vi "PV Software IGN State.vi"(11 "HEX Data (U8)":u8 format="%x") -> (3 "IGN State":string)   [LabVIEW 2023]
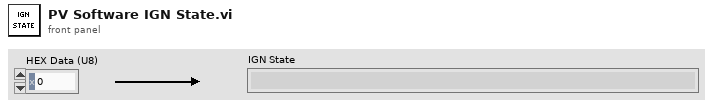
[diagram p1: front panel]
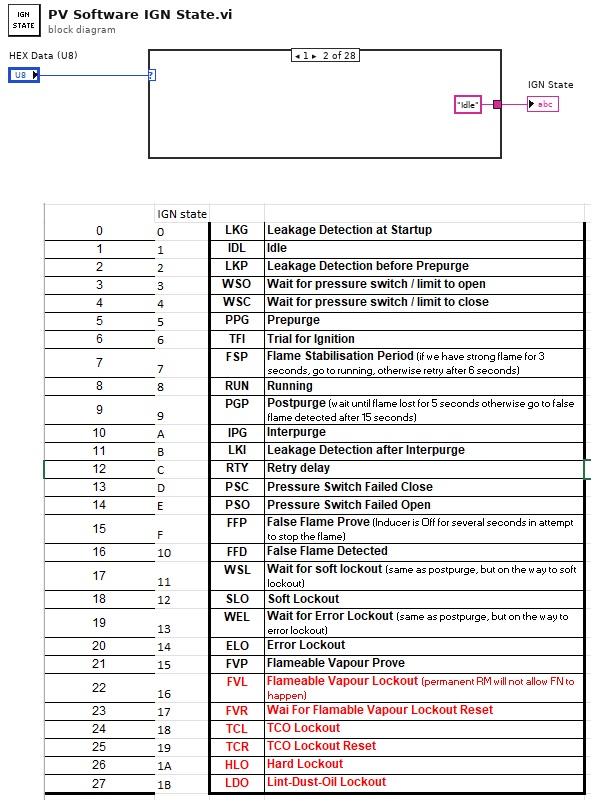
[diagram p0: block diagram]
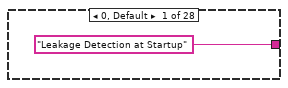
[diagram p2: hidden frame]
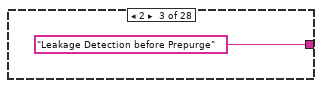
[diagram p3: hidden frame]
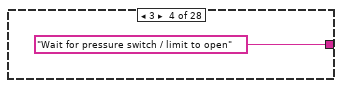
[diagram p4: hidden frame]
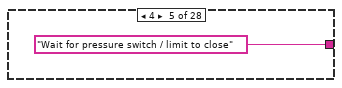
[diagram p5: hidden frame]
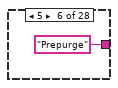
[diagram p6: hidden frame]
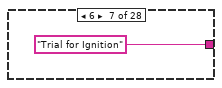
[diagram p7: hidden frame]
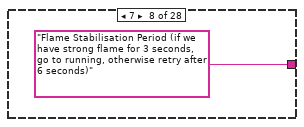
[diagram p8: hidden frame]
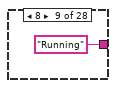
[diagram p9: hidden frame]
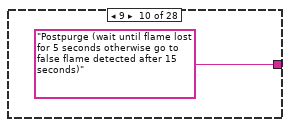
[diagram p10: hidden frame]
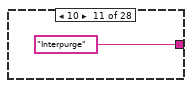
[diagram p11: hidden frame]
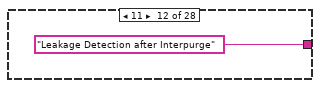
[diagram p12: hidden frame]
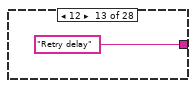
[diagram p13: hidden frame]
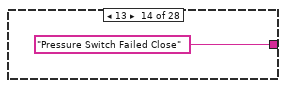
[diagram p14: hidden frame]
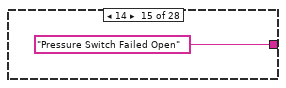
[diagram p15: hidden frame]
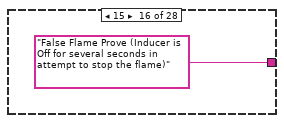
[diagram p16: hidden frame]
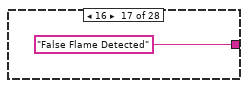
[diagram p17: hidden frame]
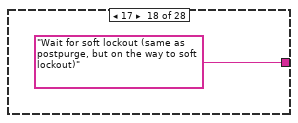
[diagram p18: hidden frame]
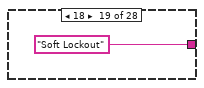
[diagram p19: hidden frame]
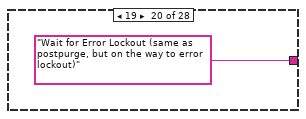
[diagram p20: hidden frame]
diagram:
  n1 = case shown="1" "HEX Data (U8)" {
    tunnel: ["Leakage Detection at Startup" "Idle" "Leakage Detection before Prepurge" "Wait for pressure switch / limit to open" "Wait for pressure switch / limit to close" "Prepurge" "Trial for Ignition" "Flame Stabilisation Period (if we have strong flame for 3 seconds, go to running, otherwise retry after 6 seconds)" "Running" "Postpurge (wait until flame lost for 5 seconds otherwise go to false flame detected after 15 seconds)" "Interpurge" "Leakage Detection after Interpurge" "Retry delay" "Pressure Switch Failed Close" "Pressure Switch Failed Open" "False Flame Prove (Inducer is Off for several seconds in attempt to stop the flame)" "False Flame Detected" "Wait for soft lockout (same as postpurge, but on the way to soft lockout)" "Soft Lockout" "Wait for Error Lockout (same as postpurge, but on the way to error lockout)" "Error Lockout" "Flameable Vapour Prove" "Flameable Vapour Lockout (permanent RM will not allow FN to happen)" "Wait For Flamable Vapour Lockout Reset" "TCO Lockout" "TCO Lockout Reset" "Hard Lockout" "Lint-Dust-Oil Lockout"] -> w1
    frame 0, Default {
    }
    frame 1 {
    }
    frame 2 {
    }
    frame 3 {
    }
    frame 4 {
    }
    frame 5 {
    }
    frame 6 {
    }
    frame 7 {
    }
    frame 8 {
    }
    frame 9 {
    }
    frame 10 {
    }
    frame 11 {
    }
    frame 12 {
    }
    frame 13 {
    }
    frame 14 {
    }
    frame 15 {
    }
    frame 16 {
    }
    frame 17 {
    }
    frame 18 {
    }
    frame 19 {
    }
    frame 20 {
    }
    frame 21 {
    }
    frame 22 {
    }
    frame 23 {
    }
    frame 24 {
    }
    frame 25 {
    }
    frame 26 {
    }
    frame 27 {
    }
  }
  "IGN State" <- w1
